vi "TA_Generate_DelayTime_LinearRandom.vi"(8 "Random\nNumber of Steps":dbl[](array[numeric])=[200.0, 200.0, 100.0, 50.0], 9 "Random \nTime Range (ps)":dbl[](array[numeric])=[1.0, 10.0, 100.0, 1000.0, 8000.0], 10 "Linear\nStep (ps)":dbl[](array[numeric])=[0.5, 0.05], 11 "Linear \nTime Range (ps)":dbl[](array[numeric])=[-10.0, -1.0, 1.0]) -> (2 "Number (Delay Time)":i32, 3 "Generated Delay Time (ps)":dbl[](array[numeric]))   [LabVIEW 2025]
uses:
  <vilib>/numeric/Random Number (Range) DBL.vi
  <vilib>/Analysis/1siggen.llb/Ramp Pattern by Delta.vi
  <vilib>/Analysis/NI_AALBase.lvlib
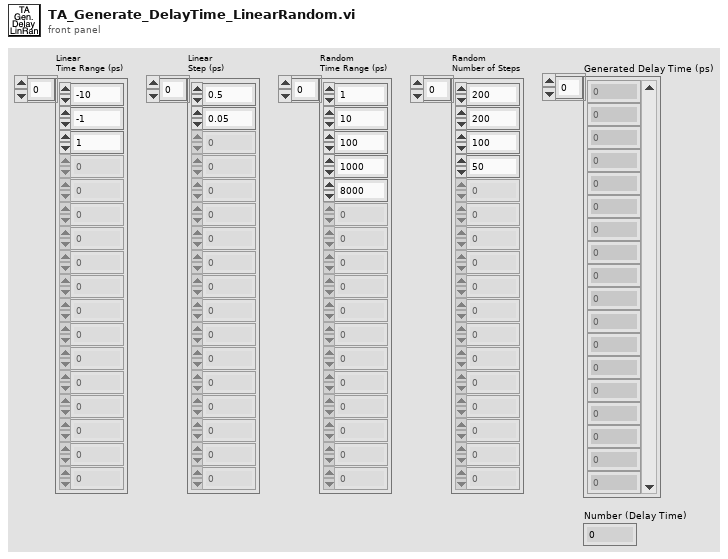
[diagram p1: front panel]
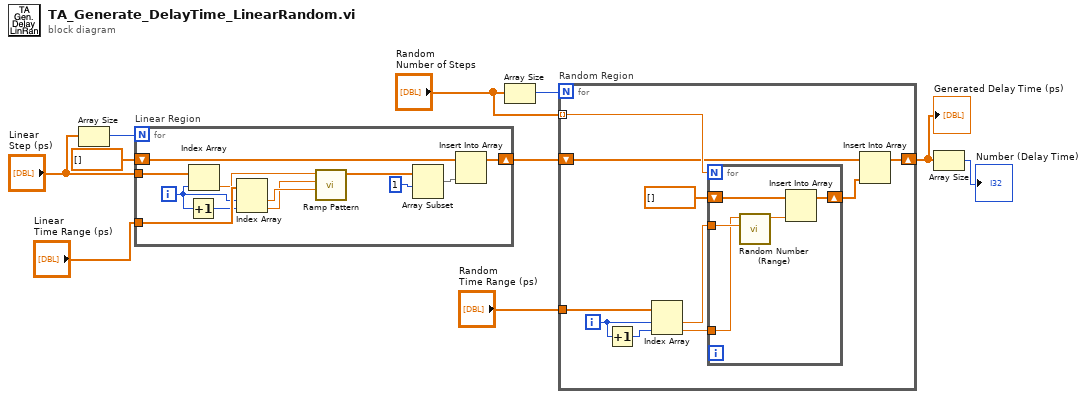
[diagram p0: block diagram]
diagram:
  n1 = Array Size(array="Linear\nStep (ps)") -> (size(s)=w9:i32)
  n2 = for "Linear Region" {
    N: w9 -> [_]
    tunnel: "Linear \nTime Range (ps)" -> [w22]
    tunnel: "Linear\nStep (ps)" -> [w18]
    shift-right: [w14] -> w2
    shift-left: dbl[] [] ("Array") -> [w15]
    i -> [w16]
    n3 = Increment(x=w16) -> (x+1=w21:i32)
    n4 = Index Array(array=w18, index=w16) -> (element=w17:dbl)
    n5 = Index Array(array=w22, index #1=w16, index #2=w21) -> (element #1=w20:dbl, element #2=w19:dbl)
    n6 = call-poly <vilib>:"Ramp Pattern.vi"("start"=w20, "end"=w19, "delta"=w17) -> ("Ramp Pattern"=w13:dbl[])  [unwired: 6 in, 2 out]
    n7 = Array Subset(array=w13, index=1) -> (w11:dbl[])  [unwired: 1 in]
    n8 = Insert Into Array(array=w15, new element=w11) -> (w14:dbl[])  [unwired: 1 in]
  }
  n9 = Array Size(array="Random\nNumber of Steps") -> (size(s)=w4:i32)
  n10 = for "Random Region" {
    N: w4 -> [_]
    tunnel: "Random \nTime Range (ps)" -> [w32]
    tunnel: "Random\nNumber of Steps" -> [w27] mode=indexing
    shift-right: [w25] -> w1
    shift-left: w2 -> [w26]
    i -> [w29]
    n11 = Increment(x=w29) -> (x+1=w28:i32)
    n12 = Index Array(array=w32, index #1=w29, index #2=w28) -> (element #1=w31:dbl, element #2=w30:dbl)
    n13 = for {
      N: w27 -> [_]
      tunnel: w31 -> [w37]
      tunnel: w30 -> [w36]
      shift-right: [w35] -> w23
      shift-left: dbl[] [] ("Array") -> [w34]
      n14 = call-poly <vilib>:"Random Number (Range).vi"("lower bound (0)"=w37, "upper bound (100)"=w36) -> ("number"=w33:dbl)  [unwired: 9 in]
      n15 = Insert Into Array(array=w34, new element=w33) -> (w35:dbl[])  [unwired: 1 in]
    }
    n16 = Insert Into Array(array=w26, new element=w23) -> (w25:dbl[])  [unwired: 1 in]
  }
  "Generated Delay Time (ps)" <- w1
  n17 = Array Size(array=w1) -> (size(s)=→"Number (Delay Time)":i32)
